vi "RT Loop - Analyze Acceleration_chopped_no_raw_data.vi"(7 "testing":bool, 8 "error in (no error)":errorcluster, 9 "Acceleration RT FIFO In":T1, 10 "FPGA VI Reference Out 2":refnum<k20>, 11 "Message Queue":refnum<queue>) -> (1 "Acceleration RT FIFO Out":T1)   [LabVIEW 2017]
doc: "Read and analyze acceleration waveform data from FPGA via DMA FIFO. If the acceleration is over the limit, then send the acceleration waveform data to the Log Data Loop."
uses:
  UI Error Handlers/support/Message Queue/Message Cluster.ctl
  controls/Acceleration RT FIFO Reference.ctl
  Globals/Global - All RT Loop Stop.vi
  Globals/Global - Configuration Options.vi
  <vilib>/Utility/error.llb/Error Cluster From Error Code.vi
  <vilib>/rvi/errors/niLvFpgaAdjustHostInterfaceError.vi
  <vilib>/rvi/interface/nirviMethod/nirviMethod.xnode
  <vilib>/FPGAPlugInAG/Dynamic/niLvFpga_ReadFifo_Dynamic.vi
  <vilib>/rvi/errors/niLvFpgaMergeErrorWithErrorCode.vi
  UI Error Handlers/support/Message Queue/Message Queue.lvlib
panel:
  out "x-y":u32
  out "G1 status":cluster{"G1 trigger":bool}
  out "G1 status.G1 trigger":bool
  out "sta":bool
  out "logical OR":bool
  in  "Data Rate (Hz)":dbl
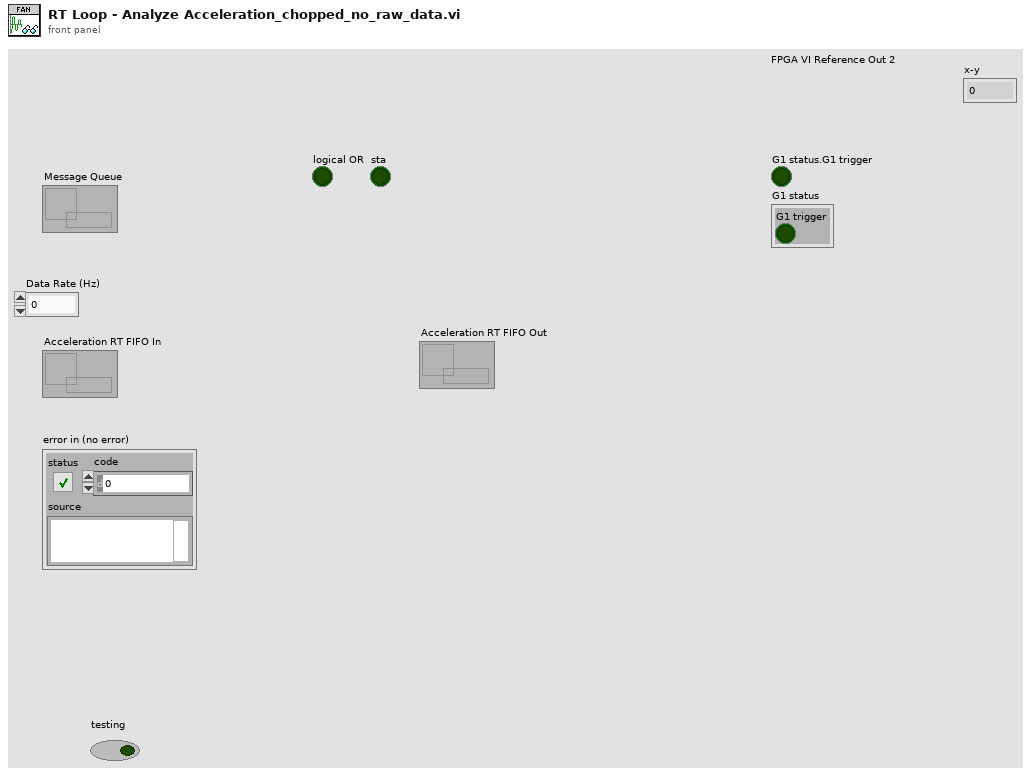
[diagram p1: front panel]
types:
  T1 = typedef "Acceleration RT FIFO Reference.ctl" = refnum<k33>
  T2 = cluster{"Tool data":cluster{"Number of teeth":sgl}, "Cutting data":cluster{"rpm":sgl}, "Limits":cluster{"Magnitude threshold":sgl, "Tolerance":sgl}, "G1 status":cluster{"G1 trigger":bool}}
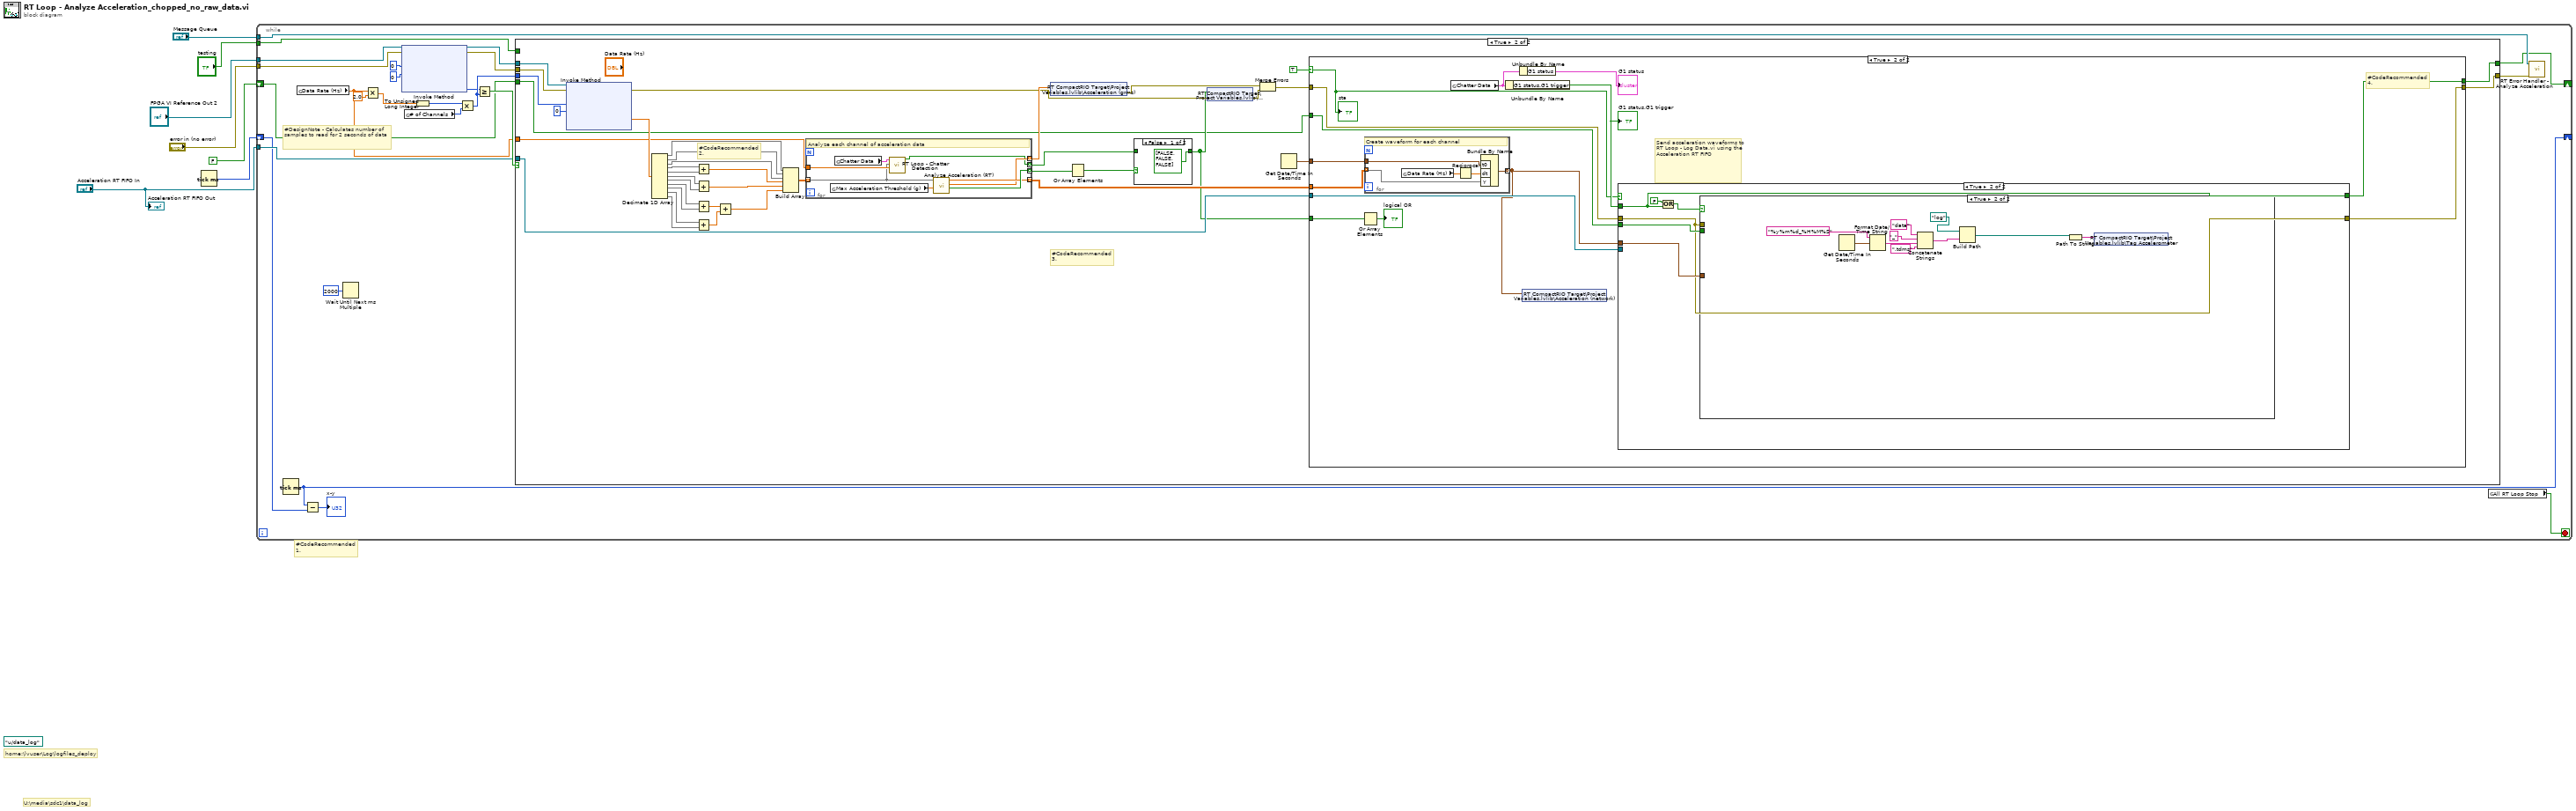
[diagram p0: block diagram]
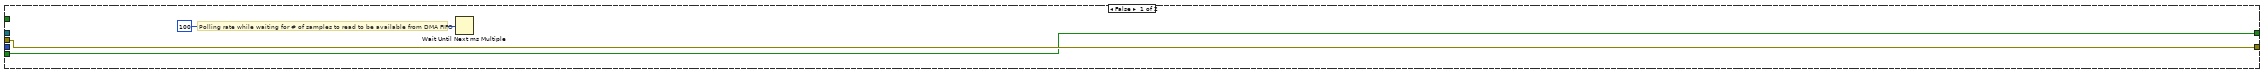
[diagram p2: hidden frame]
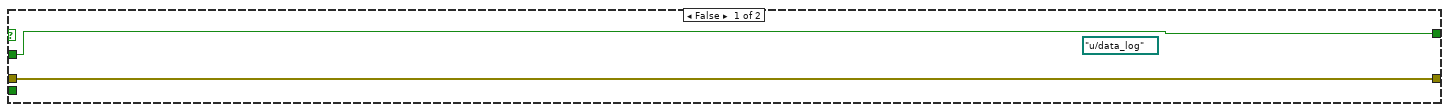
[diagram p5: hidden frame]
diagram:
  (unwired) path "u:/data_log" ("AVI Path")
  # "U:\\media\\sdc1\\data_log"
  # "home:\\lvuser\\Log\\logfiles_deploy"
  # "#CodeRecommended\n1."
  n1 = Tick Count (ms)() -> (millisecond timer value=w2:u32)
  n2 = while {
    tunnel: "FPGA VI Reference Out 2" -> [w32]
    tunnel: "error in (no error)" -> [w31]
    tunnel: "Message Queue" -> [w24]
    tunnel: "Acceleration RT FIFO In" -> [w22]
    tunnel: "testing" -> [w14]
    shift-right: [w13] -> _
    shift-left: FALSE -> [w12]
    shift-right: [w10] -> _
    shift-left: w2 -> [w11]
    stop <- w25 stop-if-true
    # "#DesignNote - Calculates number of samples to read for 2 seconds of data"
    n3 = Tick Count (ms)() -> (millisecond timer value=w10:u32)
    n4 = global read "Global - Configuration Options.vi" "Data Rate (Hz)"() -> (w16:dbl)
    n5 = Subtract(x=w10, y=w11) -> (x-y=→"x-y":u32)
    n6 = Wait Until Next ms Multiple(millisecond multiple=u32 2000) -> ()  [unwired: 1 out]
    n7 = Multiply(x=w16, y=2.0) -> (x*y=w20:dbl)
    n8 = xnode "Invoke Method"("FPGA VI Reference In"=w32, "error in"=w31, "Number of Elements"=u32 0, "Timeout (ms)"=0) -> ("FPGA VI Reference Out"=w28:refnum<k20>, "error out"=w27:errorcluster, "Elements Remaining"=w15:u32)  [unwired: 1 out]
    n9 = global read "Global - Configuration Options.vi" "# of Channels"() -> (w17:u32)
    n10 = To Unsigned Long Integer(number=w20) -> (unsigned 32bit integer=w19:u32)
    n11 = Multiply(x=w19, y=w17) -> (x*y=w18:u32)
    n12 = Greater Or Equal?(x=w15, y=w18) -> (x >= y?=w26:bool)
    n13 = case shown="True" w26 {
      tunnel: w28 -> [_ w74]
      tunnel: w27 -> [w35 w73]
      tunnel: [w35 w69] -> w23
      tunnel: w18 -> [_ w72]
      tunnel: w22 -> [_ w67]
      tunnel: w16 -> [_ w63]
      tunnel: w14 -> [_ _]
      tunnel: [w33 w55] -> w13
      tunnel: w12 -> [w33 w54]
      frame False {
        # "Polling rate while waiting for # of samples to read to be available from DMA FIFO"
        n14 = Wait Until Next ms Multiple(millisecond multiple=u32 100) -> ()  [unwired: 1 out]
      }
      frame True {
        # "#CodeRecommended\n3."
        # "#CodeRecommended\n2."
        n15 = xnode "Invoke Method"("FPGA VI Reference In"=w74, "error in"=w73, "Number of Elements"=w72, "Timeout (ms)"=0) -> ("error out"=w62:errorcluster, "Data"=w66:sgl[])  [unwired: 2 out]
        n16 = Decimate 1D Array(w66) -> (w38:sgl[], w51:sgl[], w37:sgl[], w50:sgl[], w49:sgl[], w48:sgl[], w47:sgl[], w46:sgl[], w45:sgl[], w44:sgl[], w43:sgl[])
        n17 = Add(x=w50, y=w49) -> (x+y=w36:sgl[])
        n18 = Add(x=w48, y=w47) -> (x+y=w39:sgl[])
        n19 = Add(x=w46, y=w45) -> (x+y=w42:sgl[])
        n20 = Add(x=w44, y=w43) -> (x+y=w41:sgl[])
        n21 = Add(x=w42, y=w41) -> (x+y=w40:sgl[])
        n22 = Build Array(w38, w51, w37, w36, w39, w40) -> (w52:sgl[][])
        n23 = for {
          tunnel: [w84] -> w68 mode=indexing
          tunnel: [w83] -> w65 mode=indexing
          tunnel: [w82] -> w64 mode=indexing
          tunnel: w63 -> [w80]
          tunnel: [w79] -> w57 mode=indexing
          tunnel: w52 -> [w77] mode=indexing
          # "Analyze each channel of acceleration data"
          n24 = global read "Global - Configuration Options.vi" "Max Acceleration Threshold (g)"() -> (w81:sgl)
          n25 = global read "Global - Configuration Options.vi" "Chatter Data"() -> (w78:T2)
          n26 = call "RT Loop - Chatter Detection.vi"("Data Rate (Hz)"=w80, "Acceleration Waveform (SGL)"=w77, "Chatter Data"=w78) -> ("Chatter?"=w79:bool)  [unwired: 8 in]
          n27 = call "Analyze Acceleration (RT).vi"("Max Instantaneous Acceleration (g)"=w81, "Acceleration Waveform (SGL)"=w77) -> ("Over Limit?"=w84:bool, "Acceleration (grms)"=w82:dbl, "Acceleration Waveform (DBL)"=w83:dbl[])  [unwired: 7 in]
        }
        n28 = shared-variable "RT CompactRIO Target\\Project Variables.lvlib\\Acceleration (grms)"(w64, error in=w62) -> (error out=w60:errorcluster)
        n29 = Or Array Elements(Boolean array=w68) -> (logical OR=w58:bool)
        n30 = case shown="False" w58 {
          tunnel: w57 -> [_ w76]
          tunnel: [bool[] [FALSE, FALSE, FALSE] ("Chatter?") w76] -> w56
          frame False {
          }
          frame True {
          }
        }
        n31 = shared-variable "RT CompactRIO Target\\Project Variables.lvlib\\Chatter?"(w56, error in=w62) -> (error out=w61:errorcluster)
        n32 = Merge Errors(w60, w61) -> (w59:errorcluster)
        n33 = Get Date/Time In Seconds() -> (seconds since 1Jan1904=w70:timestamp)
        n34 = case shown="True" TRUE {
          selector: TRUE -> [_ w88]
          tunnel: w70 -> [_ w100]
          tunnel: w59 -> [w86 w99]
          tunnel: [w86 w89] -> w69
          tunnel: w67 -> [_ w98]
          tunnel: w65 -> [_ w97]
          tunnel: w56 -> [_ w95]
          tunnel: [w85 w92] -> w55
          tunnel: w54 -> [w85 w91]
          frame False {
          }
          frame True {
            # "#CodeRecommended\n4."
            # "Send acceleration waveforms to RT Loop - Log Data.vi using the Acceleration RT FIFO"
            n35 = Or Array Elements(Boolean array=w95) -> (logical OR=→"logical OR":bool)
            n36 = for {
              tunnel: w97 -> [w123] mode=indexing
              tunnel: w100 -> [w122]
              tunnel: [w120] -> w87 mode=indexing
              # "Create waveform for each channel"
              n37 = global read "Global - Configuration Options.vi" "Data Rate (Hz)"() -> (w119:dbl)
              n38 = Reciprocal(x=w119) -> (1/x=w121:dbl)
              n39 = Bundle By Name("t0"=w122, "dt"=w121, "Y"=w123) -> (w120:waveform(dbl))  [unwired: 1 in]
            }
            n40 = global read "Global - Configuration Options.vi" "Chatter Data"() -> (w94:T2)
            n41 = Unbundle By Name(w94) -> ("G1 status.G1 trigger"=w90:bool)
            "G1 status.G1 trigger" <- w90
            n42 = Unbundle By Name(w94) -> ("G1 status"=→"G1 status":cluster{"G1 trigger":bool})
            n43 = shared-variable "RT CompactRIO Target\\Project Variables.lvlib\\Acceleration (network)"(w87) -> ()  [unwired: 1 in, 1 out]
            n44 = case shown="True" w88 {
              tunnel: w99 -> [w102 w103]
              tunnel: w87 -> [_ w104]
              tunnel: w98 -> [_ _]
              tunnel: w90 -> [w101 w106]
              tunnel: [w101 w106] -> w92
              tunnel: w91 -> [_ w105]
              tunnel: [w102 w103] -> w89
              frame False {
                (unwired) path "u:/data_log" ("AVI Path")
              }
              frame True {
                n45 = Or(x=FALSE, y=w106) -> (x .or. y?=w108:bool)
                n46 = case shown="True" w108 {
                  tunnel: w105 -> [_ _]
                  tunnel: w104 -> [_ _]
                  tunnel: w103 -> [_ _]
                  frame False {
                  }
                  frame True {
                    n47 = Get Date/Time In Seconds() -> (seconds since 1Jan1904=w116:timestamp)
                    n48 = Format Date/Time String(time format string (%c)="%y%m%d_%H%M%S", seconds (now)=w116) -> (date/time string=w115:string)  [unwired: 1 out]
                    n49 = Concatenate Strings("data" ("string"), "_" ("string"), w115, ".tdms" ("string")) -> (w117:string)
                    n50 = Build Path(base path=path "log", name or relative path=w117) -> (appended path=w109:path)
                    n51 = Path To String(path=w109) -> (string=w118:string)
                    n52 = shared-variable "RT CompactRIO Target\\Project Variables.lvlib\\Tag Accelerometer"(w118) -> ()  [unwired: 1 in, 1 out]
                  }
                }
              }
            }
            "sta" <- w88
          }
        }
      }
    }
    n53 = global read "Global - All RT Loop Stop.vi" "All RT Loop Stop"() -> (w25:bool)
    n54 = call "RT Error Handler - Analyze Acceleration.vi"("error in (no error)"=w23, "Message Queue"=w24) -> ()  [unwired: 9 in, 1 out]
  }
  "Acceleration RT FIFO Out" <- "Acceleration RT FIFO In"
